vi "Auto 5.vi"(8 "Error In":errorcluster) -> (0 "Error Out":errorcluster)   [LabVIEW 2014]
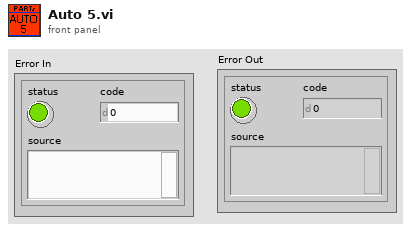
[diagram p1: front panel]
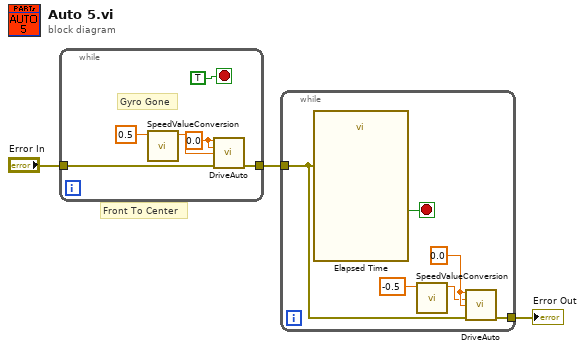
[diagram p0: block diagram]
diagram:
  # "Front To Center"
  n1 = while {
    tunnel: "Error In" -> [w9]
    tunnel: [w8] -> w3
    stop <- TRUE stop-if-true
    w7 = 0.0 ("Arm Value")
    # "Gyro Gone"
    n2 = call "SpeedValueConversion.vi"("Motor Value In"=0.5 ("X In")) -> ("New to Old Conversion Value Out"=w5:dbl)  [unwired: 9 in, 1 out]
    n3 = call "DriveAuto.vi"("X In"=w7, "Y In"=w7, "R In"=w5, "Error In"=w9) -> ("Error Out"=w8:errorcluster)  [unwired: 11 in]
  }
  n4 = while {
    tunnel: w3 -> [w12]
    tunnel: [w15] -> w2
    stop <- w13 stop-if-true
    w14 = 0.0 ("Arm Value")
    n5 = call "Elapsed Time"("error in (no error)"=w12) -> ("Time has Elapsed"=w13:bool)  [unwired: 11 in, 7 out]
    n6 = call "SpeedValueConversion.vi"("Motor Value In"=-0.5 ("X In")) -> ("New to Old Conversion Value Out"=w10:dbl)  [unwired: 9 in, 1 out]
    n7 = call "DriveAuto.vi"("X In"=w14, "Y In"=w10, "R In"=w14, "Error In"=w12) -> ("Error Out"=w15:errorcluster)  [unwired: 11 in]
  }
  "Error Out" <- w2
